vi "getSubArray2D.vi"(8 "error in (no error)":errorcluster, 9 "Index Array Cluster":T1, 10 "2D Array":dbl[][](array[numeric]), 11 "MatOper in":refnum<class "MatOper.lvclass">) -> (0 "error out":errorcluster, 2 "Sub-Array":dbl[][](array[numeric]), 3 "MatOper out":refnum<class "MatOper.lvclass">)   [LabVIEW 2016, in "MatOper.lvclass"]
doc: "Get the sub-array of the specific 2D array based on the index arrays."
uses:
  MatOper.lvclass
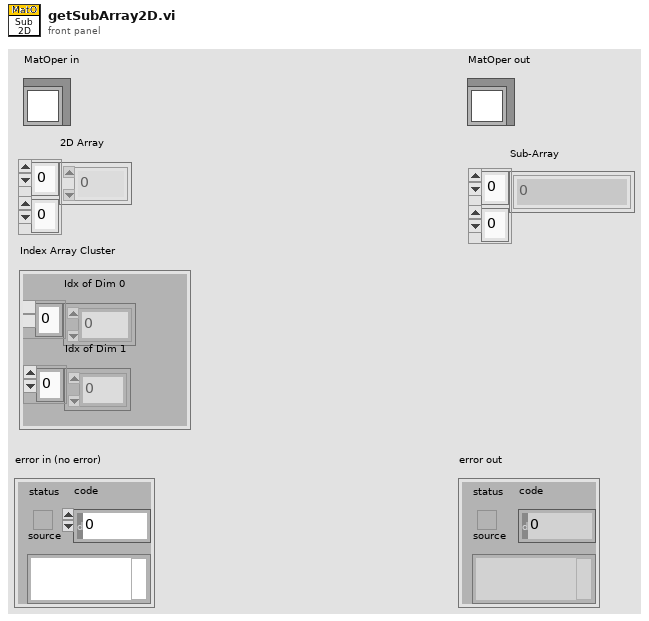
[diagram p1: front panel]
types:
  T1 = cluster{"Idx of Dim 0":i32[], "Idx of Dim 1":i32[]}
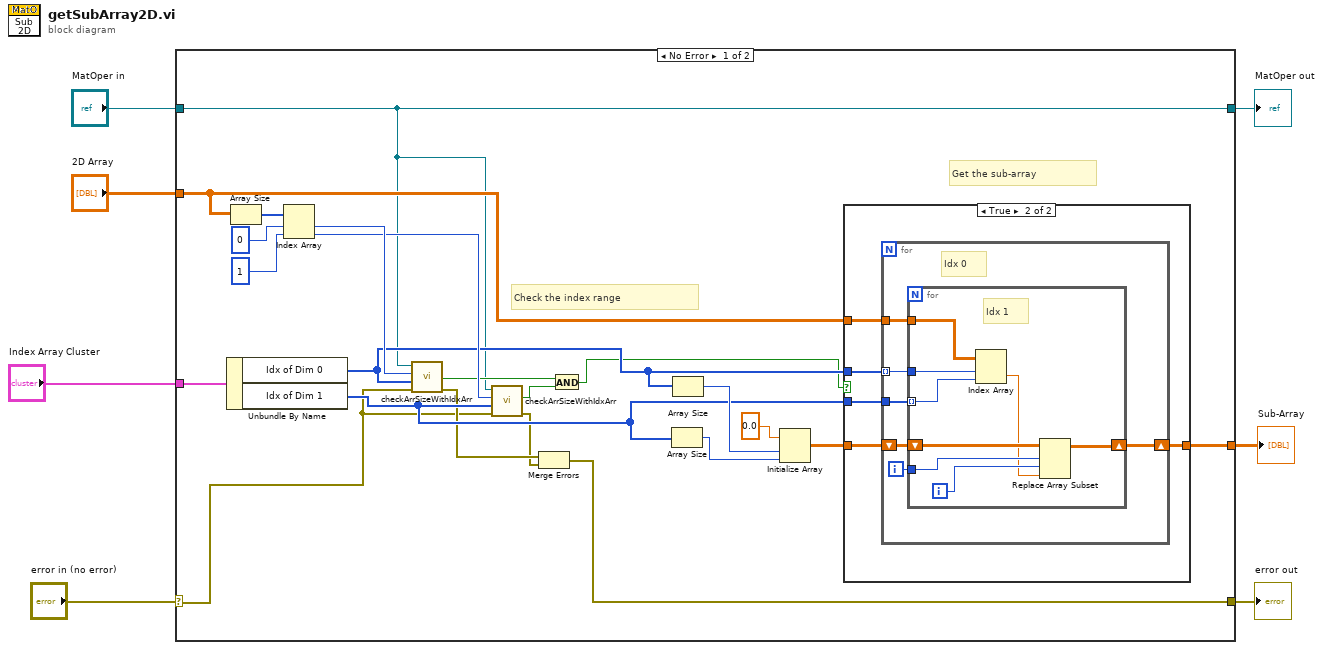
[diagram p0: block diagram]
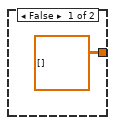
[diagram p2: hidden frame]
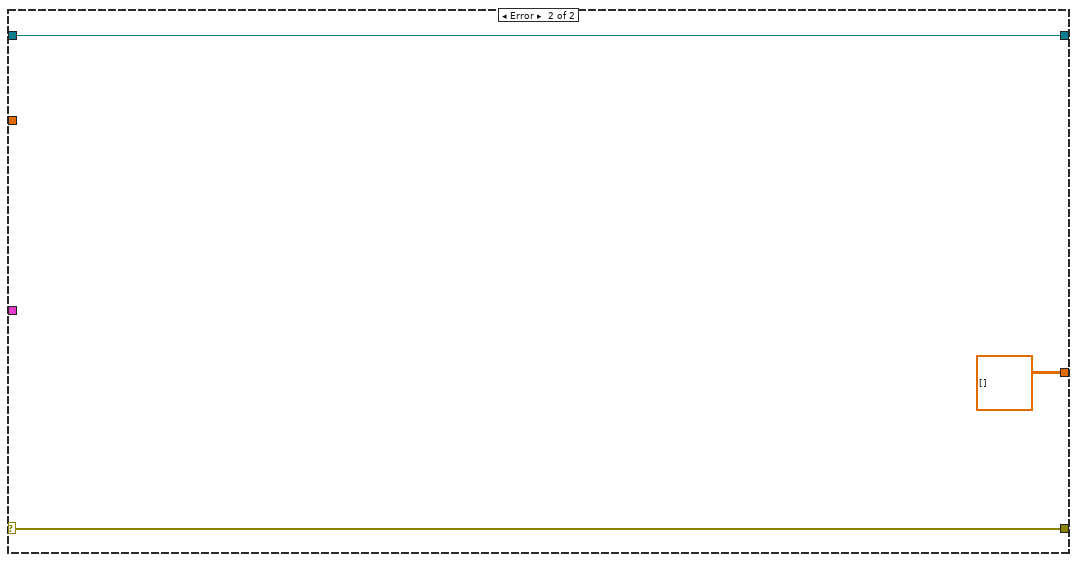
[diagram p3: hidden frame]
diagram:
  n1 = case shown="No Error" "error in (no error)" {
    selector: "error in (no error)" -> [w10 w52]
    tunnel: [w9 w52] -> w6
    tunnel: [w8 w51] -> w4
    tunnel: "MatOper in" -> [w8 w51]
    tunnel: "2D Array" -> [w13 _]
    tunnel: "Index Array Cluster" -> [w12 _]
    tunnel: [w11 dbl[][] []] -> w1
    frame No Error {
      # "Check the index range"
      # "Get the sub-array"
      n2 = Unbundle By Name(w12) -> ("Idx of Dim 0"=w18:i32[], "Idx of Dim 1"=w17:i32[])
      n3 = Array Size(array=w13) -> (size(s)=w25:i32[])
      n4 = Index Array(array=w25, index #1=0 ("index"), index #2=1 ("index")) -> (element #1=w22:i32, element #2=w21:i32)
      n5 = call "checkArrSizeWithIdxArr.vi"("error in (no error)"=w10, "Idx Array"=w18, "Array Size"=w22, "MatOper in"=w8) -> ("error out"=w15:errorcluster, "In Spec"=w20:bool)  [unwired: 5 in, 1 out]
      n6 = call "checkArrSizeWithIdxArr.vi"("error in (no error)"=w10, "Idx Array"=w17, "Array Size"=w21, "MatOper in"=w8) -> ("error out"=w14:errorcluster, "In Spec"=w19:bool)  [unwired: 5 in, 1 out]
      n7 = Merge Errors(w15, w14) -> (w9:errorcluster)
      n8 = And(x=w20, y=w19) -> (x .and. y?=w16:bool)
      n9 = Array Size(array=w17) -> (size(s)=w26:i32)
      n10 = Array Size(array=w18) -> (size(s)=w27:i32)
      n11 = Initialize Array(0.0 ("element"), w27, w26) -> (w28:dbl[][])
      n12 = case shown="True" w16 {
        tunnel: w28 -> [_ w35]
        tunnel: [dbl[][] [] w34] -> w11
        tunnel: w13 -> [_ w33]
        tunnel: w18 -> [_ w32]
        tunnel: w17 -> [_ w31]
        frame False {
        }
        frame True {
          n13 = for {
            shift-right: [w37] -> w34
            shift-left: w35 -> [w38]
            tunnel: w32 -> [w41] mode=indexing
            tunnel: w31 -> [w40]
            tunnel: w33 -> [w39]
            i -> [w36]
            # "Idx 0"
            n14 = for {
              shift-right: [w45] -> w37
              shift-left: w38 -> [w46]
              tunnel: w41 -> [w48]
              tunnel: w40 -> [w47] mode=indexing
              tunnel: w39 -> [w49]
              tunnel: w36 -> [w44]
              i -> [w43]
              # "Idx 1"
              n15 = Index Array(array=w49, index (row)=w48, index (col)=w47) -> (element=w42:dbl)
              n16 = Replace Array Subset(array=w46, new element=w42, index (row)=w44, index (col)=w43) -> (w45:dbl[][])
            }
          }
        }
      }
    }
    frame Error {
    }
  }
  "error out" <- w6
  "MatOper out" <- w4
  "Sub-Array" <- w1
